vi "test_Add Waveform Output Channels.vi"(8 "error in (no error)":errorcluster, 11 "TestCase in":refnum<class "FPGA Addon Adding a Channel Item.lvclass">) -> (0 "error out":errorcluster, 3 "TestCase out":refnum<class "FPGA Addon Adding a Channel Item.lvclass">)   [LabVIEW 2019, in "FPGA Addon Adding a Channel Item.lvclass"]
uses:
  FPGA Addon Adding a Channel Item.lvclass
  <vilib>/NI VeriStand/Custom Device API/Custom Device Channel.ctl
  <vilib>/NI VeriStand/Custom Device API/Custom Device Channel Type.ctl
  Addon/Addon System Explorer/Types/Channel Type.ctl
  Addon/Addon Shared/Types/FG Action.ctl
  FPGA Addon Adding a Channel Item.lvclass/FPGA Addon Adding a Channel Item.ctl
  Addon/Addon Shared/SubVIs/Constants.vi
  <vilib>/NI VeriStand/Custom Device Tools/Custom Device Utility Library/NI VeriStand - Search for Item by GUID.vi
  <vilib>/NI/NI VeriStand Advanced SysDef API/SysDef API/SysDef.Property.Get.vi
  <vilib>/NI/NI VeriStand Advanced SysDef API/_SubVIs/SysDef.Property.Get.Variant.vi
  <vilib>/NI/NI VeriStand Advanced SysDef API/SysDef API/SysDef.Property.Set.vi
  <vilib>/NI/NI VeriStand Advanced SysDef API/_SubVIs/SysDef.Property.Set.Variant.vi
  <vilib>/NI/NI VeriStand Advanced SysDef API/_SubVIs/SysDef.Search.GUIDs.vi
  <vilib>/addons/_JKI Toolkits/VI Tester/TestCase.llb/TestCase.lvclass
  Addon/Addon System Explorer/FPGA Addon System Explorer.lvlib
  Addon/Addon Shared/FPGA Addon Shared.lvlib
  <vilib>/NI VeriStand/Custom Device Tools/Custom Device Utility Library/Custom Device Utility Library.lvlib
  <vilib>/NI/NI VeriStand Advanced SysDef API/SysDef API/Advanced System Definition.lvlib
  <vilib>/NI VeriStand/Custom Device API/Custom Device API.lvlib
  C:/Program Files (x86)/National Instruments/LabVIEW 2019/vi.lib/addons/_JKI Toolkits/VI Tester/TestCase.llb/TestCase.lvclass
panel:
  out "GUIDs":string[](array[string])
  out "Channels":T1[](array[typedef])
  in  "remove":bool
  in  "add":bool
  out "Names":string[](array[string])
  in  "Available Registers":i32[](listbox)
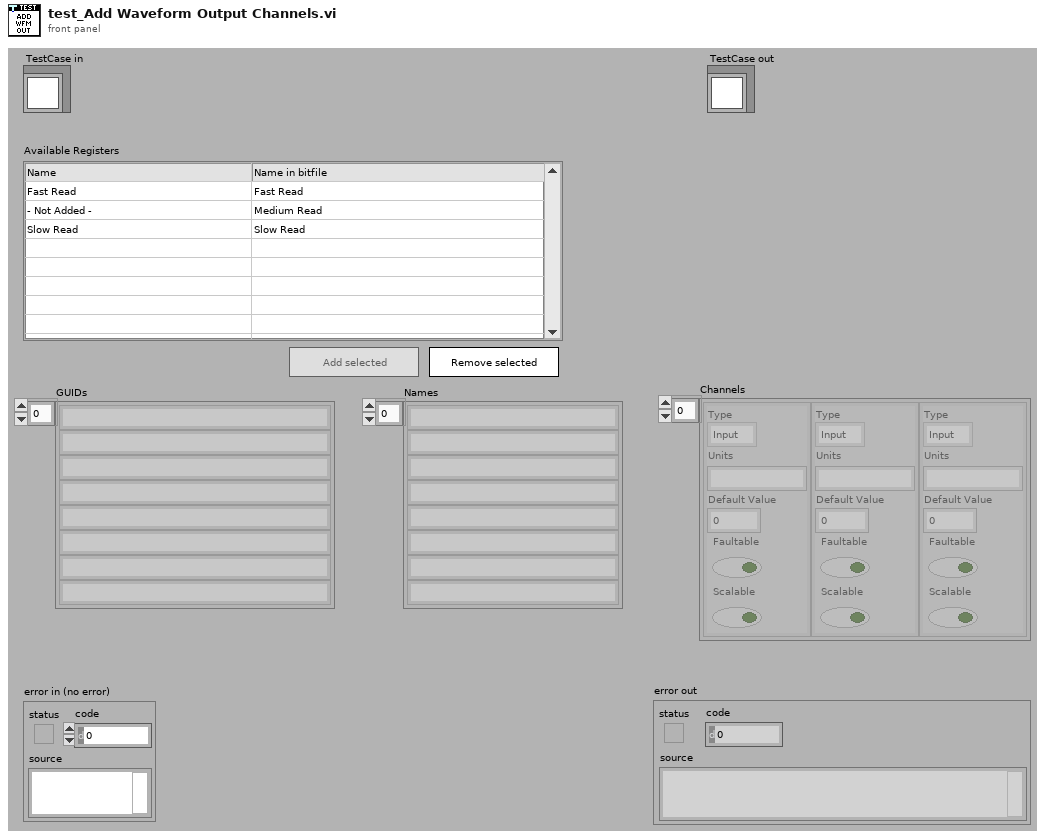
[diagram p1: front panel]
types:
  T1 = typedef "Custom Device API.lvlib/Custom Device Channel.ctl" = cluster{"Type":T2, "Units":string, "Default Value":dbl, "Faultable":bool, "Scalable":bool}
  T2 = typedef "Custom Device API.lvlib/Custom Device Channel Type.ctl" = enum16{"Input", "Output"}
  T3 = typedef "FPGA Addon Shared.lvlib/FG Action.ctl" = enum8{"GET", "SET"}
  T4 = typedef "FPGA Addon System Explorer.lvlib/Channel Type.ctl" = enum16{"Write Channel", "Read Channel", "Write Waveform", "Read Waveform"}
  T5 = typedef "Custom Device API.lvlib/Custom Device Item Ref.ctl" = u64
  T6 = typedef "FPGA Addon Shared.lvlib/DMA Information.ctl" = cluster{"Name":string, "Data Type":T7}
  T7 = typedef "FPGA Addon Shared.lvlib/Data Type.ctl" = enum8{"<Null>", "I8", "I16", "I32", "I64", "U8", "U16", "U32", "U64", "SGL", "Boolean", "Analog PWM In Settings", "Analog PWM In", "Digital PWM In Settings", "Digital PWM In", "Digital PWM Out", "Sine Out", "FXP+/-24.5", "FXP+/-16.5", "FXP+/-32.8", "FXP+/-64.32", "FXP+/-16.7", "FXP+/-20.5", "FXP+/-27.5", "FXP+/-32.16", "FXP+16.3", "FXP+18.3", "Digital Static In", "Digital Static Out", "Digital Static In Settings", "Digital WSS Out", "Quad Encoder Settings", "Quad Encoder In", "Group"}
  T8 = typedef "FPGA Addon System Explorer.lvlib/Listbox Cluster.ctl" = cluster{"add":refnum<vi>, "remove":refnum<vi>, "Listbox":refnum<vi>, "selected":i32[], "not present":i32[], "listbox text":string[][], "Section Ref":T5}
  T9 = typedef "Advanced System Definition.lvlib/TreeItem.Info.ctl" = cluster{"Name":string, "Description":string, "GUID":string, "Is Channel":bool, "Channel":T1, "Is Waveform":bool, "Waveform":T10}
  T10 = typedef "Custom Device API.lvlib/Custom Device Waveform.ctl" = cluster{"Data Type":T11, "Units":string}
  T11 = typedef "Custom Device API.lvlib/Custom Device Waveform DataType.ctl" = enum16{"Double", "Complex Double"}
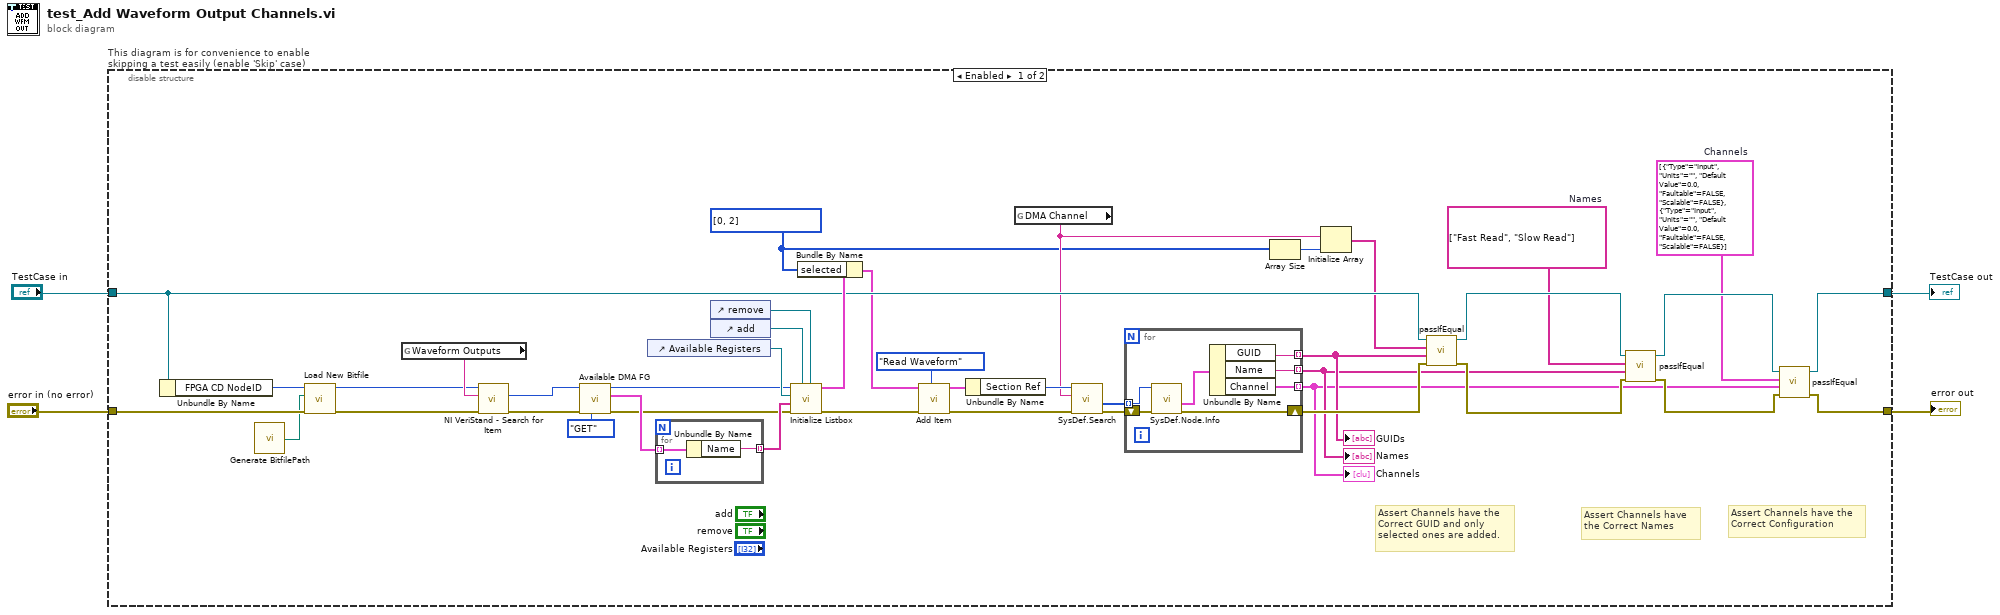
[diagram p0: block diagram]
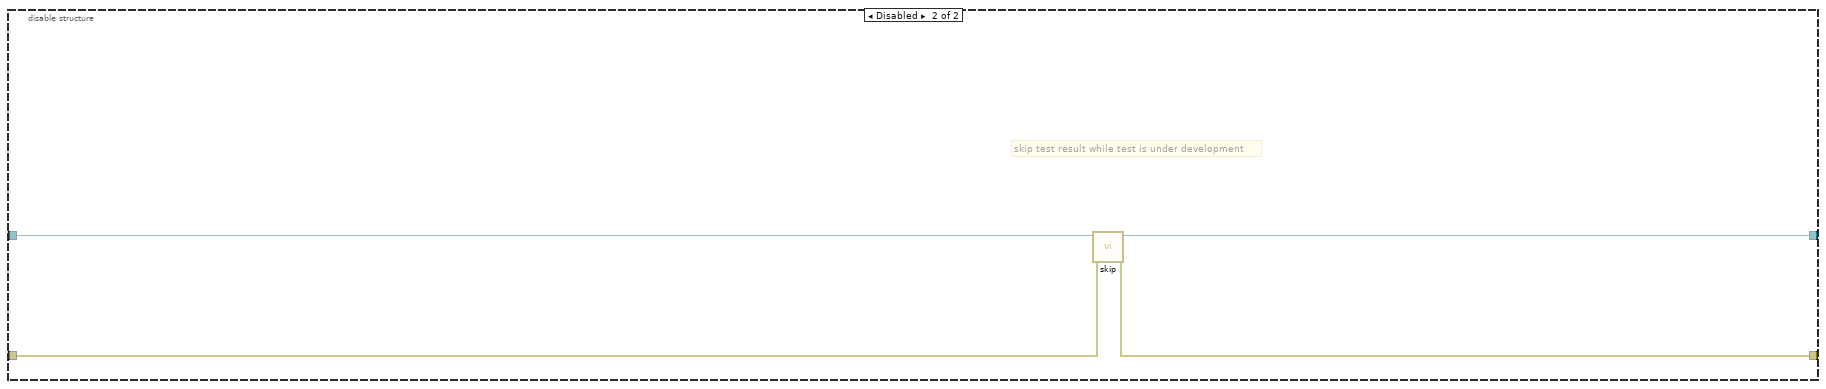
[diagram p2: hidden frame]
diagram:
  n1 = disable-structure "This diagram is for convenience to enable skipping a test easily (enable 'Skip' case)" shown="Enabled" {
    disable-tunnel: "TestCase in" -> [w32 w59]
    disable-tunnel: [w28 w57] -> w1
    disable-tunnel: [w25 w58] -> w3
    disable-tunnel: "error in (no error)" -> [w22 w56]
    frame Enabled {
      w24 = T1[] [{"Type"=enum."Input", "Units"="", "Default Value"=0.0, "Faultable"=FALSE, "Scalable"=FALSE}, {"Type"=enum."Input", "Units"="", "Default Value"=0.0, "Faultable"=FALSE, "Scalable"=FALSE}]  # Channels
      w29 = string[] ["Fast Read", "Slow Read"]  # Names
      w15 = i32[] [0, 2] ("selected")
      # "Assert Channels have the Correct Configuration"
      # "Assert Channels have the Correct Names"
      # "Assert Channels have the Correct GUID and only selected ones are added."
      n2 = Unbundle By Name(w32) -> ("FPGA CD NodeID"=w21:u64)
      n3 = call "Generate BitfilePath.vi"() -> ("Bitfile path"=w20:path)
      n4 = call "Load New Bitfile.vi"("error in (no error)"=w22, "NewVal"=w20, "Item Ref in"=w21) -> ("error out"=w23:errorcluster, "Section Ref out"=w13:T5)  [unwired: 7 in]
      n5 = global read "Constants.vi" "Waveform Outputs"() -> (w42:string)
      n6 = call-poly <vilib>:"NI VeriStand - Search for Item.vi"("error in"=w23, "Item GUID"=w42, "Section Ref in"=w13) -> ("error out"=w10:errorcluster, "Item Ref"=w11:T5)  [unwired: 5 in, 2 out]
      n7 = call "Available DMA FG.vi"("Action"=FG_Action."GET", "error in (no error)"=w10, "Item Ref"=w11) -> ("error out"=w7:errorcluster, "Available DMA"=w8:T6[], "Item Ref out"=w9:T5)  [unwired: 6 in]
      n8 = control-ref of="Available Registers"() -> (w46:refnum<vi>)
      n9 = for {
        tunnel: w8 -> [w48] mode=indexing
        tunnel: [w47] -> w45 mode=indexing
        n10 = Unbundle By Name(w48) -> ("Name"=w47:string)
      }
      n11 = control-ref of="remove"() -> (w37:refnum<vi>)
      n12 = control-ref of="add"() -> (w38:refnum<vi>)
      n13 = call "Initialize Listbox.vi"("remove"=w37, "add"=w38, "error in (no error)"=w7, "Names"=w45, "Listbox"=w46, "Item Ref"=w9) -> ("error out"=w41:errorcluster, "Listbox Refs"=w43:T8)  [unwired: 4 in]
      n14 = Bundle By Name(cluster=w43, "selected"=w15) -> (w19:T8)
      n15 = call "Add Item.vi"("Action"=Channel_Type."Read Waveform", "error in (no error)"=w41, "Listbox Refs in"=w19) -> ("error out"=w6:errorcluster, "Listbox Refs out"=w18:T8)  [unwired: 7 in]
      n16 = Unbundle By Name(w18) -> ("Section Ref"=w39:T5)
      n17 = global read "Constants.vi" "DMA Channel"() -> (w16:string)
      n18 = call-poly <vilib>:"SysDef.Search.vi"("error in (no error)"=w6, "GUID"=w16, "nodeID"=w39) -> ("error out"=w40:errorcluster, "Values Out"=w36:u64[])  [unwired: 5 in, 2 out]
      n19 = for {
        tunnel: w36 -> [w52] mode=indexing
        tunnel: [w50] -> w30 mode=indexing
        tunnel: [w49] -> w5 mode=indexing
        tunnel: [w51] -> w33 mode=indexing
        shift-right: [w54] -> w34
        shift-left: w40 -> [w55]
        n20 = call <vilib>:"SysDef.Node.Info.vi"("error in (no error)"=w55, "nodeID"=w52) -> ("error out"=w54:errorcluster, "Item Info"=w53:T9)  [unwired: 6 in, 2 out]
        n21 = Unbundle By Name(w53) -> ("GUID"=w51:string, "Name"=w50:string, "Channel"=w49:T1)
      }
      "Names" <- w30
      "Channels" <- w5
      "GUIDs" <- w33
      n22 = Array Size(array=w15) -> (size(s)=w14:i32)
      n23 = Initialize Array(w16, w14) -> (w17:string[])
      n24 = call-dynamic "passIfEqual.vi"("error in (no error)"=w34, "y"=w33, "x"=w17, "TestCase in"=w32) -> ("error out"=w35:errorcluster, "TestCase out"=w31:refnum<class "FPGA Addon Adding a Channel Item.lvclass">)  [unwired: 6 in]
      n25 = call-dynamic "passIfEqual.vi"("error in (no error)"=w35, "y"=w30, "x"=w29, "TestCase in"=w31) -> ("error out"=w26:errorcluster, "TestCase out"=w27:refnum<class "FPGA Addon Adding a Channel Item.lvclass">)  [unwired: 6 in]
      n26 = call-dynamic "passIfEqual.vi"("error in (no error)"=w26, "y"=w5, "x"=w24, "TestCase in"=w27) -> ("error out"=w25:errorcluster, "TestCase out"=w28:refnum<class "FPGA Addon Adding a Channel Item.lvclass">)  [unwired: 6 in]
    }
    frame Disabled {
      # "skip test result while test is under development"
      n27 = call <vilib>:"skip.vi"("error in (no error)"=w56, "TestCase in"=w59) -> ("error out"=w58:errorcluster, "TestCase out"=w57:refnum<class "FPGA Addon Adding a Channel Item.lvclass">)  [unwired: 8 in]
    }
  }
  "error out" <- w3
  "TestCase out" <- w1
